vi "is visible to load.vi"(8 "error in":errorcluster, 11 "TBM Configuration Node in":refnum<class "TBM Configuration Node.lvclass">) -> (0 "error out":errorcluster, 2 "visible":bool, 3 "TBM Configuration Node out":refnum<class "TBM Configuration Node.lvclass">)   [LabVIEW 2013, in "PL Framework Configuration Tool.lvlib" / "TBM Configuration Node.lvclass"]
doc: "Determines whether a node should be visible when generating right click menus. By default, any abstract node is not visible."
uses:
  TBM Configuration Node.lvclass
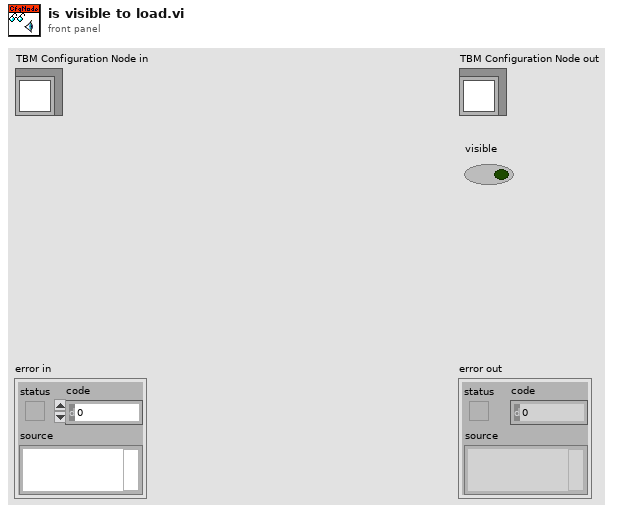
[diagram p1: front panel]
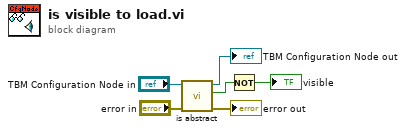
[diagram p0: block diagram]
diagram:
  n1 = call-dynamic "is abstract.vi"("error in"="error in", "NISE_CEF_serializable node in"="TBM Configuration Node in") -> ("error out"=→"error out":errorcluster, "abstract"=w2:bool, "NISE_CEF_serializable node out"=→"TBM Configuration Node out":refnum<class "TBM Configuration Node.lvclass">)  [unwired: 7 in]
  n2 = Not(x=w2) -> (.not. x?=→"visible":bool)
